vi "Reserve (Poly).vi"   [LabVIEW 2020, in "Measurement Service Helpers.lvlib"]
doc: "Reserves sessions based on the provided pin information."
uses:
  Measurement Service Helpers.lvlib
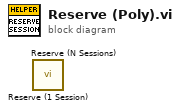
[diagram p0: block diagram]
diagram:
  n1 = call "Reserve (1 Session).vi"() -> ()  [unwired: 8 in, 4 out]
  n2 = call "Reserve (N Sessions).vi"() -> ()  [unwired: 8 in, 4 out]
